vi "LimeSDR_BandWidth_Tx_LabVIEW_V1.1.vi"() -> ()   [LabVIEW 2018, in "LMS_LV_Drv.lvlib"]
uses:
  LMS_LV_Drv.lvlib
  <vilib>/addons/Modulation/Digital/Support/Common/Validators/mod_AWGN Validate.vi
  <vilib>/addons/Modulation/Analog/support/mod_Set Error Source.vi
  <vilib>/addons/Modulation/Digital/Impairments/subVIs/mod_createSeeds.vi
  <vilib>/addons/Modulation/Digital/Impairments/subVIs/mod_IQ Impairments Gain Imbalance.vi
  <vilib>/addons/Modulation/Digital/Impairments/subVIs/mod_IQ Impairments Quadrature Skew.vi
  <vilib>/addons/Modulation/Digital/Impairments/subVIs/mod_IQ Impairments Axis Shear.vi
  <vilib>/addons/Modulation/Digital/Impairments/subVIs/mod_IQ Impairments DC Offset.vi
  <vilib>/addons/Modulation/Digital/Impairments/subVIs/mod_IQ Impairments Frequency Offset.vi
  <vilib>/addons/Modulation/Digital/Support/Common/Validators/mod_Validate Samples Per Symbol.vi
  <vilib>/addons/Modulation/Analog/support/Validators/mod_Validate Complex Waveform.vi
  <vilib>/Analysis/5stat.llb/RMS.vi
  <vilib>/Analysis/5stat.llb/RMS (DBL).vi
  <vilib>/addons/Modulation/Digital/Support/Common/mod_Apply Frequency Offset.vi
  <vilib>/addons/Modulation/Analog/support/Validators/mod_WFErrorHandler.vi
  <vilib>/addons/Modulation/Digital/Support/Common/mod_Apply Frequency Offset (Internal).vi
  <vilib>/addons/Modulation/Digital/General/subVIs/mod_Generate Bits PN Sequence.vi
  <vilib>/Analysis/1siggen.llb/Gaussian White Noise (obs 90).vi
  <vilib>/addons/Modulation/Digital/Support/Common/Validators/mod_IQ Impairments Validate.vi
  <vilib>/addons/Modulation/niDMT.lvlib
panel:
  out "Y":cdb[](array[numeric])
  in  "Reset":bool=TRUE
  in  "Eb/N0, dB":dbl(slide)=40.0 scale=0.0..100.0
  in  "TX Filter":T1(ring)=enum."Raised Cosine"
  in  "M-QAM":T2(ring)=enum."16"
  in  "Symbol Rate":dbl=1000000.0 step=1000.0 format="%.2p"
  in  "# Message Symbols":i32=1000
  in  "Frequency Offset, Hz":dbl(slide) scale=-1000.0..1000.0
  out "unsigned 64bit integer":u64=20981760
  in  "Boolean":bool
  out "Numeric":i32=77836066
  out "return":i32=2098176
  in  "Direction":u8(ring) items=["RX", "TX"]
  out "EXIT":bool=TRUE
  in  "stop":bool
  in  "FM  Frequency":dbl(slide)=500000000.0 min=85000000.0 max=108000000.0 step=50000.0 scale=85000000.0..108000000.0 scale format="%#_6p"
  in  "chan":u64
  out "LimeSDR_info":string="LimeSDR-USB, media=USB 3.0, module=FX3, serial=0009072C02891115, index=0"
  in  "Sample Rate":dbl=2000000.0 format="%#_6p"
  out "error out":errorcluster
  # "Two Tone Generation Demo"
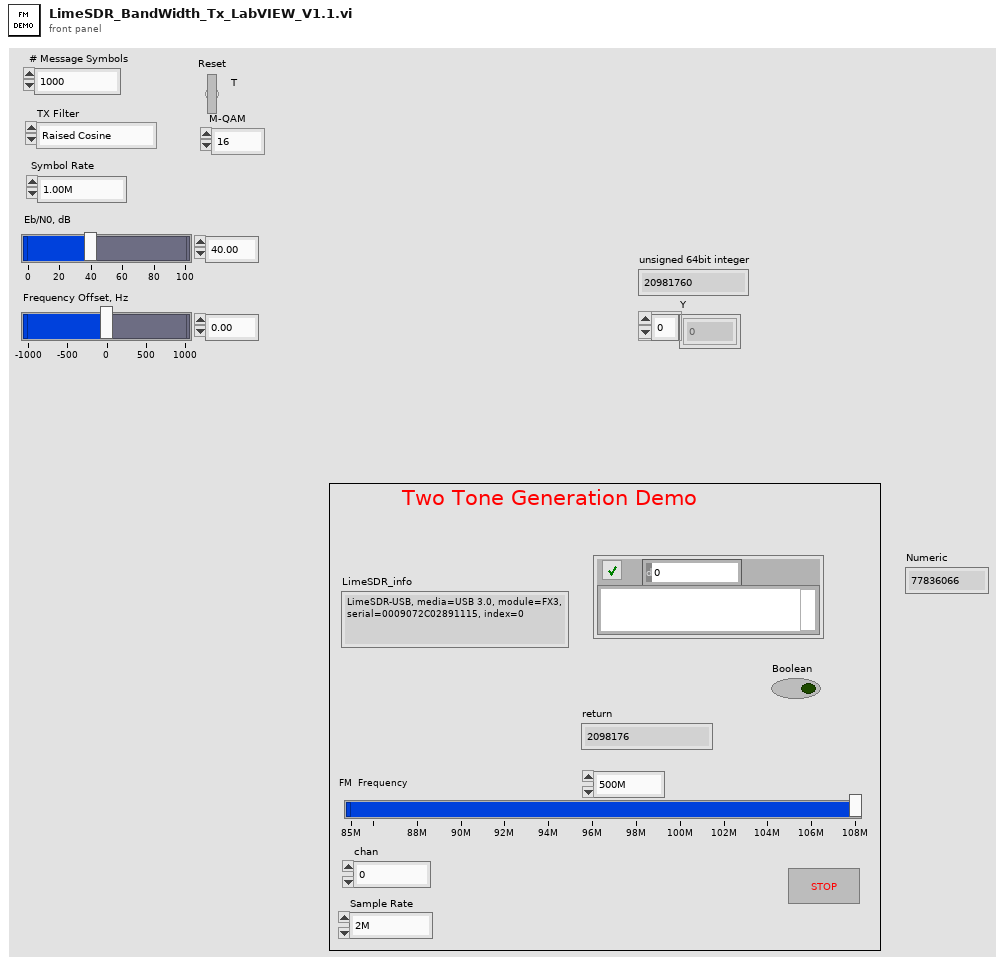
[diagram p1: front panel]
types:
  T1 = enum16{"none", "Raised Cosine", "Root Raised Cos", "Gaussian"}
  T2 = enum16{"4", "8", "16", "32", "64", "128", "256", "512", "1024", "2048", "4096"}
  T3 = cluster{"# Guard Bits":i32, "# Sync Bits":i32, "# Message Bits":i32, "PN sequence order":i32}
  T4 = cluster{"TX Filter":enum16{"none", "Raised Cosine", "Root Raised Cos", "Gaussian"}, "filter parameter":dbl, "filter length":i32}
  T5 = typedef "niAMT.lvlib/Complex Data Waveform.ctl" = cluster{"t0":dbl, "dt":dbl, "Y":cdb[]}
  T6 = typedef "niDMT.lvlib/QAM System Parameters.ctl" = cluster{"samples per symbol (16)":i32, "symbol map":cdb[]}
  T7 = cluster{"Output Bit Stream":i8[], " # bits per symbol":i32, "Sync (Bits)":i8[], "Sync (Symbols)":cdb[], "pulse shaping filter coefficients":dbl[], "matched filter coefficients":dbl[], "QAM System Parameters":T6}
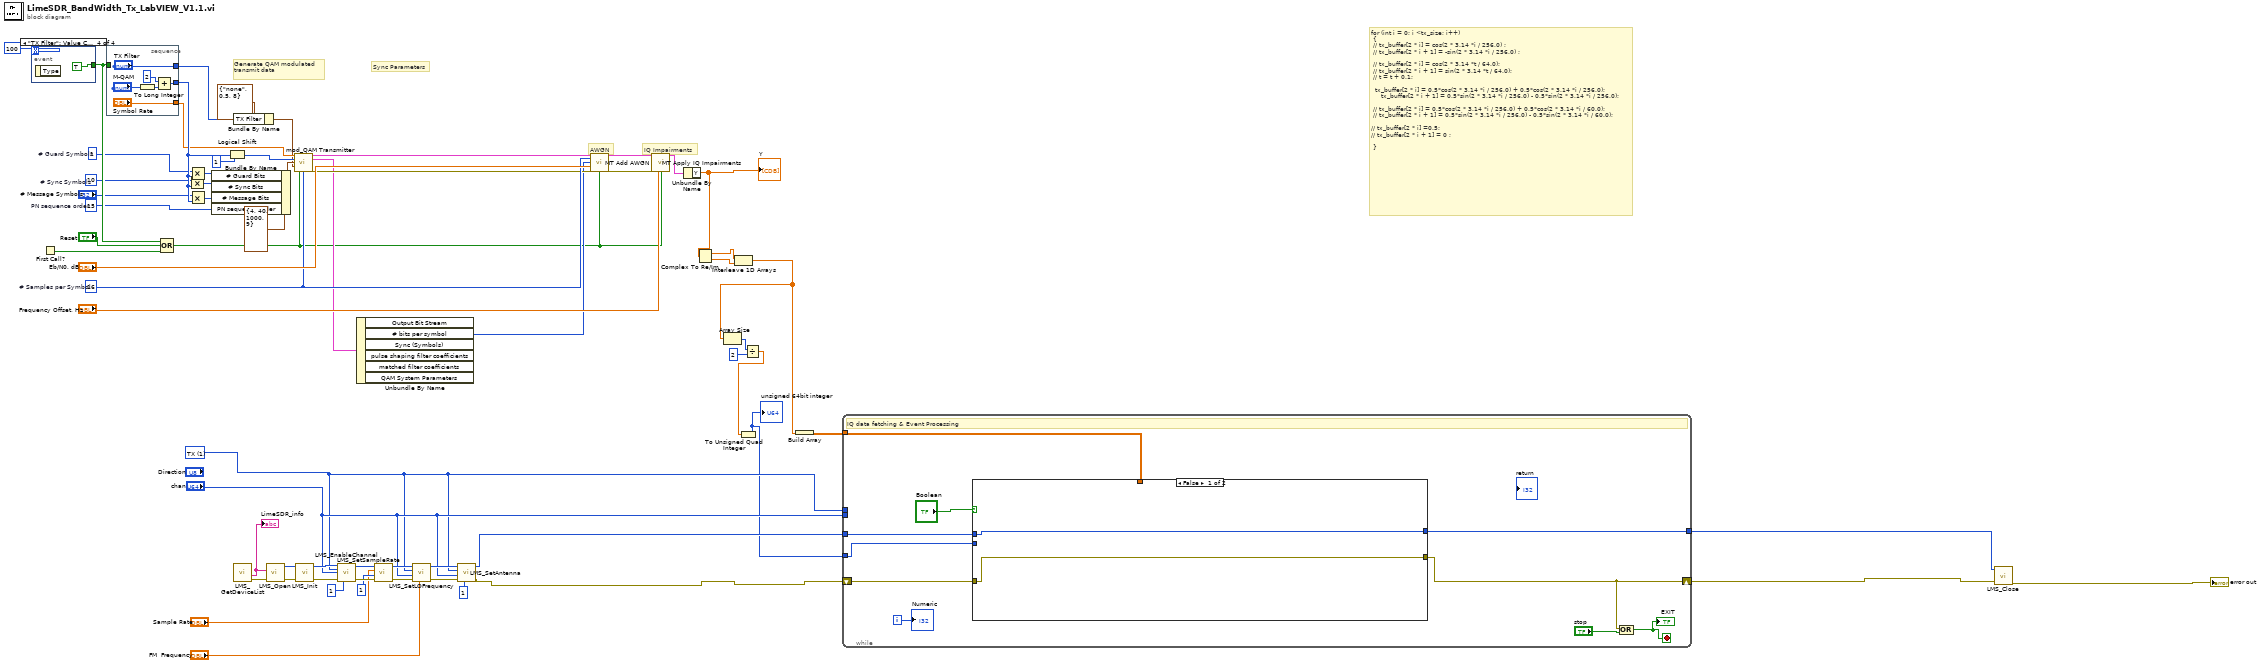
[diagram p0: block diagram]
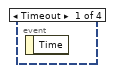
[diagram p2: hidden frame]
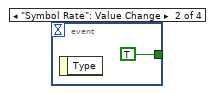
[diagram p3: hidden frame]
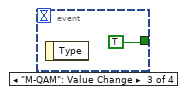
[diagram p4: hidden frame]
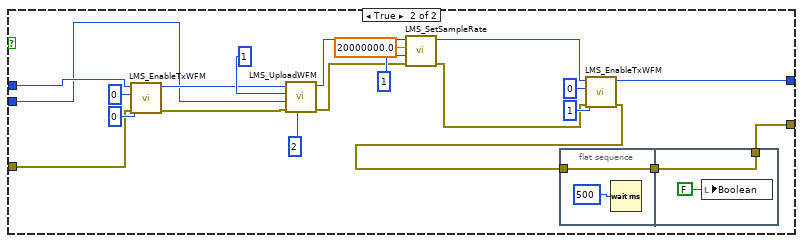
[diagram p5: hidden frame]
diagram:
  w15 = 15  # PN sequence order
  w20 = 16  # # Samples per Symbol
  w30 = 10  # # Sync Symbols
  w13 = 1  # # Guard Symbols
  w47 = u8 1 items=["RX", "TX"] ("Direction")
  # "IQ Impairments"
  # "Sync Parameters"
  # "Generate QAM modulated\ntransmit data"
  # "AWGN"
  # "for (int i = 0; i <tx_size; i++)\n\t{\n\t//\ttx_buffer[2 * i] = cos(2 * 3.14 *i / 256.0) ;\n\t//\ttx_buffer[2 * i + 1] = -sin(2 * 3.14 *i / 256.0) ;\n\n\t//\ttx_buffer[2 * i] = cos(2 * 3.14 *t / 64.0);\n\t//\ttx_buffer[2 * i + 1] = sin(2 * 3.14 *t / 64.0);\n\t//\tt = t + 0.1;\n\n\t\ttx_buffer[2 * i] = 0.5*cos(2 * 3.14 *i / 256.0) + 0.5*cos(2 * 3.14 *i / 256.0);\n    \ttx_buffer[2 * i + 1] = 0.5*sin(2 * 3.14 *i / 256.0) - 0.5*sin(2 * 3.14 *i / 256.0);\n\n\t//\ttx_buffer[2 * i] = 0.5*cos(2 * 3.14 *i / 256.0) + 0.5*cos(2 * 3.14 *i / 60.0);\n\t//\ttx_buffer[2 * i + 1] = 0.5*sin(2 * 3.14 *i / 256.0) - 0.5*sin(2 * 3.14 *i / 60.0);\n\n//\ttx_buffer[2 * i] =0.5;\n//\ttx_buffer[2 * i + 1] = 0 ;\n\n\t}"
  n1 = event shown="[3] \"TX Filter\": Value Change" {
    selector: _ -> [_ _ _ _]
    dyn-events: _ -> [_ _ _ _]
    timeout: 100 -> [_ _ _ _]
    tunnel: [_ TRUE TRUE TRUE] -> w35
    event Timeout {
      n2 = event-data() -> ()  [unwired: 1 in, 1 out]
    }
    event "Symbol Rate": Value Change {
      n3 = event-data() -> ()  [unwired: 1 in, 1 out]
    }
    event "M-QAM": Value Change {
      n4 = event-data() -> ()  [unwired: 1 in, 1 out]
    }
    event "TX Filter": Value Change {
      n5 = event-data() -> ()  [unwired: 1 in, 1 out]
    }
  }
  n6 = First Call?() -> (First Call?: T/F=w36:bool)
  n7 = stacked-sequence {
    tunnel: w35 -> [_]
    tunnel: ["TX Filter"] -> w17
    tunnel: [w71] -> w31
    tunnel: ["Symbol Rate"] -> w21
    frame #0 {
      n8 = To Long Integer(number="M-QAM") -> (32bit integer=w70:i32)
      n9 = Add(x=2, y=w70) -> (x+y=w71:i32)
    }
  }
  n10 = Compound Arithmetic op=OR(w35, "Reset", w36) -> (w10:bool)
  n11 = Multiply(x=w30, y=w31) -> (x*y=w29:i32)
  n12 = Multiply(x=w13, y=w31) -> (x*y=w26:i32)
  n13 = Multiply(x="# Message Symbols", y=w31) -> (x*y=w28:i32)
  n14 = Bundle By Name(cluster=T3 {"# Guard Bits"=4, "# Sync Bits"=40, "# Message Bits"=1000, "PN sequence order"=9} ("Message"), "# Guard Bits"=w26, "# Sync Bits"=w29, "# Message Bits"=w28, "PN sequence order"=w15) -> (w27:T3)
  n15 = Logical Shift(y=w31, x=1) -> (x << y=w33:i32)
  n16 = Bundle By Name(cluster=T4 {"TX Filter"=enum."none", "filter parameter"=0.5, "filter length"=8} ("System Filter"), "TX Filter"=w17) -> (w16:T4)
  n17 = call "LMS_GetDeviceList.vi"() -> ("error out"=w64:errorcluster, "lms_info_str_t"=w63:string)  [unwired: 9 in, 1 out]
  "LimeSDR_info" <- w63
  n18 = call "LMS_Open.vi"("error in (no error)"=w64, "lms_info_str_t"=w63) -> ("error out"=w62:errorcluster, "device"=w61:i64)  [unwired: 8 in]
  n19 = call <vilib>:"mod_QAM Transmitter.vi"("Symbol Rate, Hz"=w21, "Reset?"=w10, "# Samples per Symbol"=w20, "M-QAM"=w33, "Message"=w27, "System Filter"=w16) -> ("Output Complex Waveform"=w19:T5, "Signal Description"=w12:T7, "error out"=w14:errorcluster)  [unwired: 7 in]
  n20 = call "LMS_Init.vi"("error in (no error)"=w62, "device_In"=w61) -> ("error out"=w59:errorcluster, "device_Out"=w60:i64)  [unwired: 8 in]
  n21 = call "LMS_EnableChannel.vi"("device_In"=w60, "dir_tx"=w47, "chan"="chan", "error in (no error)"=w59, "enabled"=i8 1) -> ("device_Out"=w56:i64, "error out"=w57:errorcluster)  [unwired: 9 in]
  n22 = Unbundle By Name(w12) -> ("# bits per symbol"=w11:i32)  [unwired: 5 out]
  n23 = call "LMS_SetSampleRate.vi"("error in (no error)"=w57, "oversample"=u64 1, "rate"="Sample Rate", "device_In"=w56) -> ("error out"=w55:errorcluster, "device_Out"=w54:i64)  [unwired: 6 in]
  n24 = call "LMS_SetLOFrequency.vi"("frequency"="FM  Frequency", "error in (no error)"=w55, "chan"="chan", "dir_tx"=w47, "device_In"=w54) -> ("error out"=w52:errorcluster, "device_Out"=w51:i64)  [unwired: 5 in]
  n25 = call "LMS_SetAntenna.vi"("index"=u64 1, "error in (no error)"=w52, "chan"="chan", "dir_tx"=w47, "device_In"=w51) -> ("error out"=w44:errorcluster, "device_Out"=w42:i64)  [unwired: 5 in]
  n26 = call <vilib>:"MT Add AWGN.vi"("input complex waveform"=w19, "samples per symbol (16)"=w20, "bits per symbol (1)"=w11, "Eb/N0 (10 dB)"="Eb/N0, dB", "error in (no error)"=w14, "reset? (T)"=w10) -> ("output complex waveform"=w24:T5, "error out"=w23:errorcluster)  [unwired: 7 in, 1 out]
  n27 = call <vilib>:"MT Apply IQ Impairments.vi"("input complex waveform"=w24, "error in (no error)"=w23, "frequency offset (Hz)"="Frequency Offset, Hz", "reset? (T)"=w10) -> ("output complex waveform"=w9:T5)  [unwired: 10 in, 1 out]
  n28 = Unbundle By Name(w9) -> ("Y"=w6:cdb[])
  "Y" <- w6
  n29 = Complex To Re/Im(x + iy=w6) -> (x=w8:dbl[], y=w7:dbl[])
  n30 = Interleave 1D Arrays(w8, w7) -> (w5:dbl[])
  n31 = Array Size(array=w5) -> (size(s)=w4:i32)
  n32 = Divide(x=w4, y=2) -> (x/y=w2:dbl)
  n33 = To Unsigned Quad Integer(1:w2) -> (0:w1:u64)
  "unsigned 64bit integer" <- w1
  n34 = Build Array(w5) -> (w40:dbl[][])
  n35 = while {
    shift-right: [w79] -> w43
    shift-left: w44 -> [w80]
    tunnel: w47 -> [_]
    tunnel: "chan" -> [_]
    tunnel: w1 -> [w75]
    tunnel: w42 -> [w78]
    tunnel: [w77] -> w41
    tunnel: w40 -> [w76]
    i -> [w81]
    stop <- w83 stop-if-true
    # "IQ data fetching & Event Processing"
    n36 = case shown="False" "Boolean" {
      tunnel: w80 -> [w84 w96]
      tunnel: [w84 w101] -> w79
      tunnel: w78 -> [w85 w93]
      tunnel: [w85 w106] -> w77
      tunnel: w76 -> [_ _]
      tunnel: w75 -> [_ w92]
      frame False {
      }
      frame True {
        n37 = call "LMS_EnableTxWFM.vi"("error in (no error)"=w96, "active"=i8 0, "chan"=u64 0, "device_In"=w93) -> ("error out"=w95:errorcluster, "device_Out"=w94:i64)  [unwired: 6 in]
        n38 = call "LMS_UploadWFM.vi"("format"=2, "error in (no error)"=w95, "sample_count"=w92, "ChannelCount"=u8 1, "Dev"=w94) -> ("error out"=w88:errorcluster, "Dev_out"=w90:i64)  [unwired: 5 in]
        n39 = call "LMS_SetSampleRate.vi"("error in (no error)"=w88, "oversample"=u64 1, "rate"=20000000.0, "device_In"=w90) -> ("error out"=w87:errorcluster, "device_Out"=w89:i64)  [unwired: 6 in]
        n40 = flat-sequence {
          tunnel: [w107] -> w100
          tunnel: w99 -> [w107]
          tunnel: [w109] -> w101
          tunnel: w100 -> [w109]
          frame #0 {
            n41 = Wait (ms)(milliseconds to wait=u32 500) -> ()  [unwired: 1 out]
          }
          frame #1 {
            n42 = local write "Boolean"(FALSE ("Boolean")) -> ()
          }
        }
        n43 = call "LMS_EnableTxWFM.vi"("error in (no error)"=w87, "active"=i8 1, "chan"=u64 0, "device_In"=w89) -> ("error out"=w99:errorcluster, "device_Out"=w106:i64)  [unwired: 6 in]
      }
    }
    n44 = Compound Arithmetic op=OR(w79, "stop") -> (w83:bool)
    "EXIT" <- w83
    "Numeric" <- w81
  }
  n45 = call "LMS_Close.vi"("error in (no error)"=w43, "device_In"=w41) -> ("error out"=→"error out":errorcluster)  [unwired: 9 in]
